vi "JSONtext Example.vi"() -> ()   [LabVIEW 2015]
uses:
  Find Object Items by Name.vi
  Find Object Items by Path.vi
  Get I32.vi
  Find Object Item (single) by Path.vi
  Get String.vi
  String Subset.vi
  support/Quote and Escape JSON string.vi
  support/Strip Quotes and Unescape.vi
  Get Number Text.vi
  Advance past String.vi
  support/quote and escape json string 2.vi
  Advance past Number.vi
  Insert into Object.vi
  JSON text to Variant.vi
  Find Item Locations by Path.vi
  support/Unescape JSON string.vi
  Parsing Error.vi
  Find Object Item Locations by Names.vi
  JSONtext.lvlib
panel:
  out "<JSON> 2":string[](array[string]) caption="Found in x object"
  in  "Pretty Print?":bool=TRUE
  out "All (incl. Added Array)":T1
  out "out":T2(array[cluster])
  out "x.inputs.prev_out.addr":string[](array[string])
  out "x.vin_sz":i32[](array[numeric])
  in  "Added Array Size":i32=10
  in  "Test Cluster":T3={"op"="utx", "x"={"lock_time"=0, "ver"=1, "size"=192, "inputs"=[{"sequence"=4294967295, "prev_out"={"spent"=TRUE, "tx_index"=99005468, "type"=0, "addr"="1BwGf3z7n2fHk6NoVJNkV32qwyAYsMhkWf", "value"=65574000, "n"=0, "script"="76a91477f4c9ee75e449a74c21a4decfb50519cbc245b388ac"}, "script"="483045022100e4ff962c292705f051c2c2fc519fa775a4d8955bce1a3e29884b2785277999ed02200b537ebd22a9f25fbbbcc9113c69c1389400703ef2017d80959ef0f1d685756c012102618e08e0c8fd4c5fe539184a30fe35a2f5fccf7ad62054cad29360d871f8187d"}, {"sequence"=22222222, "prev_out"={"spent"=TRUE, "tx_index"=99005469, "type"=1, "addr"="Blah Blah Blah", "value"=222222, "n"=0, "script"="76a91477f4c9ee75e449a74c21a4decfb50519cbc245b388ac"}, "script"="483045022100e4ff962c292705f051c2c2fc519fa775a4d8955bce1a3e29884b2785277999ed02200b537ebd22a9f25fbbbcc9113c69c1389400703ef2017d80959ef0f1d685756c012102618e08e0c8fd4c5fe539184a30fe35a2f5fccf7ad62054cad29360d871f8187d"}], "time"=1440086763, "tx_index"=99006637, "vin_sz"=1, "hash"="0857b9de1884eec314ecf67c040a2657b8e083e1f95e31d0b5ba3d328841fc7f", "vout_sz"=1, "relayed_by"="127.0.0.1", "out"=[{"spent"=FALSE, "tx_index"=99006637, "type"=0, "addr"="1A828tTnkVFJfSvLCqF42ohZ51ksS3jJgX", "value"=65564000, "n"=0, "script"="76a914640cfdf7b79d94d1c980133e3587bd6053f091f388ac"}, {"spent"=TRUE, "tx_index"=123, "type"=0, "addr"="1A828tTnkVFJfSvLCqF42ohZ51ksS3jJgX", "value"=13234312, "n"=1, "script"="76a914640cfdf7b79d94d1c980133e3587bd6053f091f388ac"}]}}
  out "<JSON>":string
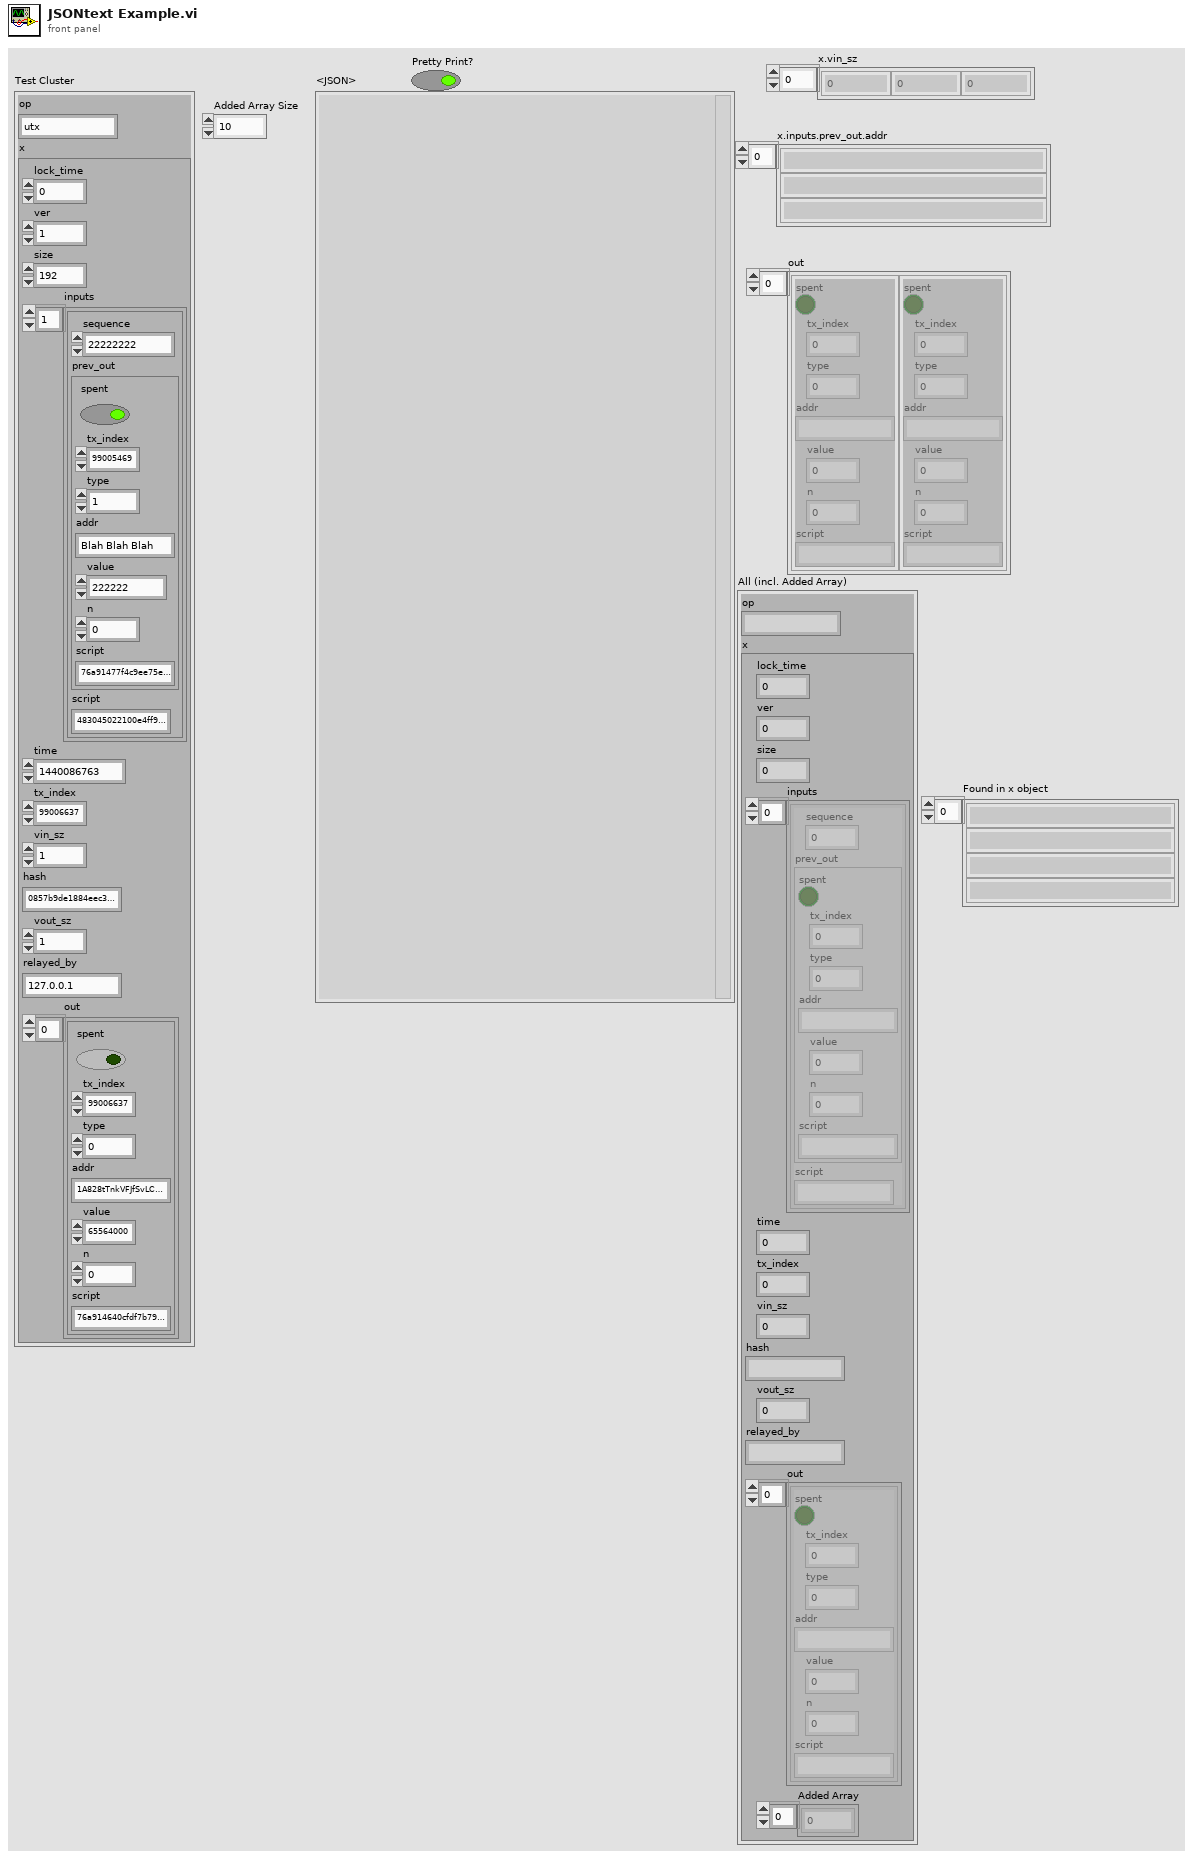
[diagram p1: front panel]
types:
  T1 = cluster{"op":string, "x":cluster{"lock_time":i32, "ver":i32, "size":i32, "inputs":cluster{"sequence":i64, "prev_out":cluster{"spent":bool, "tx_index":i32, "type":i32, "addr":string, "value":i32, "n":i32, "script":string}, "script":string}[], "time":i32, "tx_index":i32, "vin_sz":i32, "hash":string, "vout_sz":i32, "relayed_by":string, "out":cluster{"spent":bool, "tx_index":i32, "type":i32, "addr":string, "value":i32, "n":i32, "script":string}[], "Added Array":dbl[]}}
  T2 = cluster{"spent":bool, "tx_index":i32, "type":i32, "addr":string, "value":i32, "n":i32, "script":string}[]
  T3 = cluster{"op":string, "x":cluster{"lock_time":i32, "ver":i32, "size":i32, "inputs":cluster{"sequence":i64, "prev_out":cluster{"spent":bool, "tx_index":i32, "type":i32, "addr":string, "value":i32, "n":i32, "script":string}, "script":string}[], "time":i32, "tx_index":i32, "vin_sz":i32, "hash":string, "vout_sz":i32, "relayed_by":string, "out":cluster{"spent":bool, "tx_index":i32, "type":i32, "addr":string, "value":i32, "n":i32, "script":string}[]}}
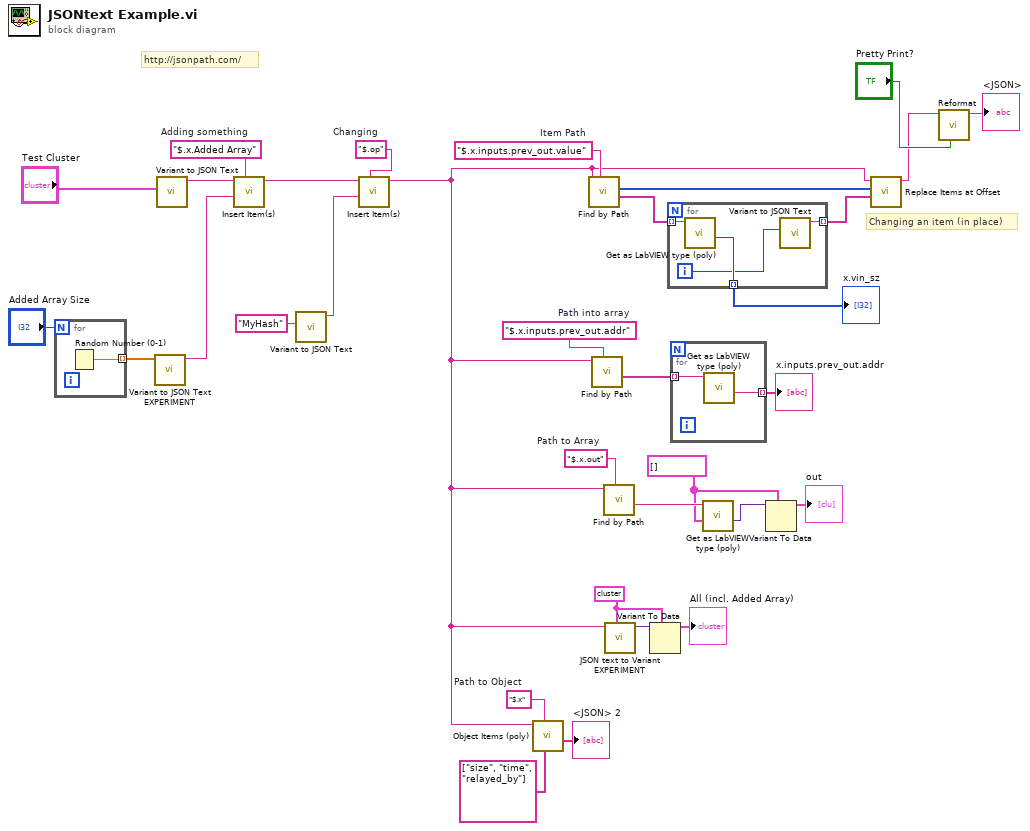
[diagram p0: block diagram]
diagram:
  w13 = "$.x"  # Path to Object
  w7 = T2 []
  w17 = "$.x.out"  # Path to Array
  w21 = "$.x.inputs.prev_out.addr"  # Path into array
  w22 = "$.x.inputs.prev_out.value"  # Item Path
  w27 = "$.op"  # Changing
  w6 = T1 {"op"="utx", "x"={"lock_time"=0, "ver"=1, "size"=192, "inputs"=[{"sequence"=4294967295, "prev_out"={"spent"=TRUE, "tx_index"=99005468, "type"=0, "addr"="1BwGf3z7n2fHk6NoVJNkV32qwyAYsMhkWf", "value"=65574000, "n"=0, "script"="76a91477f4c9ee75e449a74c21a4decfb50519cbc245b388ac"}, "script"="483045022100e4ff962c292705f051c2c2fc519fa775a4d8955bce1a3e29884b2785277999ed02200b537ebd22a9f25fbbbcc9113c69c1389400703ef2017d80959ef0f1d685756c012102618e08e0c8fd4c5fe539184a30fe35a2f5fccf7ad62054cad29360d871f8187d"}, {"sequence"=22222222, "prev_out"={"spent"=TRUE, "tx_index"=99005469, "type"=1, "addr"="Blah Blah Blah", "value"=222222, "n"=0, "script"="76a91477f4c9ee75e449a74c21a4decfb50519cbc245b388ac"}, "script"="483045022100e4ff962c292705f051c2c2fc519fa775a4d8955bce1a3e29884b2785277999ed02200b537ebd22a9f25fbbbcc9113c69c1389400703ef2017d80959ef0f1d685756c012102618e08e0c8fd4c5fe539184a30fe35a2f5fccf7ad62054cad29360d871f8187d"}], "time"=1440086763, "tx_index"=99006637, "vin_sz"=1, "hash"="0857b9de1884eec314ecf67c040a2657b8e083e1f95e31d0b5ba3d328841fc7f", "vout_sz"=1, "relayed_by"="127.0.0.1", "out"=[{"spent"=FALSE, "tx_index"=99006637, "type"=0, "addr"="1A828tTnkVFJfSvLCqF42ohZ51ksS3jJgX", "value"=65564000, "n"=0, "script"="76a914640cfdf7b79d94d1c980133e3587bd6053f091f388ac"}, {"spent"=TRUE, "tx_index"=123, "type"=0, "addr"="1A828tTnkVFJfSvLCqF42ohZ51ksS3jJgX", "value"=13234312, "n"=1, "script"="76a914640cfdf7b79d94d1c980133e3587bd6053f091f388ac"}], "Added Array"=[]}} ("Test Cluster")
  w31 = "$.x.Added Array"  # Adding something
  # "Changing an item (in place)"
  # "http://jsonpath.com/"
  n1 = for {
    N: "Added Array Size" -> [_]
    tunnel: [w34] -> w29 mode=indexing
    n2 = Random Number (0-1)() -> (number: 0 to 1=w34:dbl)
  }
  n3 = call "Variant to JSON Text EXPERIMENT.vi"("Variant"=w29) -> ("<JSON>"=w12:string)  [unwired: 9 in, 1 out]
  n4 = call "Variant to JSON Text.vi"("Variant"="Test Cluster") -> ("<JSON>"=w32:string)  [unwired: 8 in, 2 out]
  n5 = call-poly "Insert Item(s).vi"("Object (or Item) Path"=w31, "JSON to Insert"=w12, "JSON in"=w32) -> ("<JSON>"=w28:string)  [unwired: 5 in, 2 out]
  n6 = call "Variant to JSON Text.vi"("Variant"="MyHash" ("JSON to Insert")) -> ("<JSON>"=w11:string)  [unwired: 8 in, 2 out]
  n7 = call-poly "Insert Item(s).vi"("Object (or Item) Path"=w27, "JSON to Insert"=w11, "JSON in"=w28) -> ("<JSON>"=w2:string)  [unwired: 5 in, 2 out]
  n8 = call-poly "Object Items (poly).vi"("Item Names"=string[] ["size", "time", "relayed_by"], "Object Path"=w13, "JSON"=w2) -> ("<JSON>"=→"<JSON> 2":string[])  [unwired: 6 in, 2 out]
  n9 = call-poly "Find by Path.vi"("Item Path"=w22, "JSON"=w2) -> ("<JSON>"=w10:string[], "Offsets"=w5:i32[])  [unwired: 6 in, 2 out]
  n10 = call-poly "Find by Path.vi"("Item Path"=w21, "JSON"=w2) -> ("<JSON>"=w20:string[])  [unwired: 6 in, 3 out]
  n11 = call-poly "Find by Path.vi"("Item Path"=w17, "JSON"=w2) -> ("<JSON>"=w18:string)  [unwired: 6 in, 3 out]
  n12 = call "JSON text to Variant EXPERIMENT.vi"("Data Type and Default Value"=w6, "JSON"=w2) -> ("Variant out"=w9:variant)  [unwired: 8 in, 1 out]
  n13 = Variant To Data(type=w6, Variant=w9) -> (data=→"All (incl. Added Array)":T1)  [unwired: 1 in, 1 out]
  n14 = for {
    tunnel: w10 -> [w38] mode=indexing
    tunnel: [w37] -> w4 mode=indexing
    tunnel: [w36] -> w3 mode=indexing
    i -> [w35]
    n15 = call-poly "Get as LabVIEW type (poly).vi"("JSON"=w38) -> ("Number"=w37:i32)  [unwired: 9 in, 1 out]
    n16 = call "Variant to JSON Text.vi"("Variant"=w35) -> ("<JSON>"=w36:string)  [unwired: 8 in, 2 out]
  }
  "x.vin_sz" <- w4
  n17 = for {
    tunnel: w20 -> [w40] mode=indexing
    tunnel: [w39] -> w19 mode=indexing
    n18 = call-poly "Get as LabVIEW type (poly).vi"("JSON"=w40) -> ("String"=w39:string)  [unwired: 8 in, 2 out]
  }
  "x.inputs.prev_out.addr" <- w19
  n19 = call-poly "Get as LabVIEW type (poly).vi"("Data Type"=w7, "JSON"=w18) -> ("Variant out"=w8:variant)  [unwired: 8 in, 1 out]
  n20 = Variant To Data(type=w7, Variant=w8) -> (data=→"out":T2)  [unwired: 1 in, 1 out]
  n21 = call "Replace Items at Offset.vi"("<JSON>New Items"=w3, "Offsets of Item to Replace"=w5, "<JSON> in"=w2) -> ("<JSON>"=w1:string)  [unwired: 8 in]
  n22 = call "Reformat.vi"("Pretty Print?"="Pretty Print?", "JSON"=w1) -> ("<JSON>"=→"<JSON>":string)  [unwired: 6 in, 2 out]
